vi "temporisador.vi"() -> ()   [LabVIEW 2020]
panel:
  in  "Auto Reset":bool=TRUE
  in  "Time Target (s)":dbl=1.0
  out "Numeric":i32
  in  "stop":bool
  in  "reset":bool
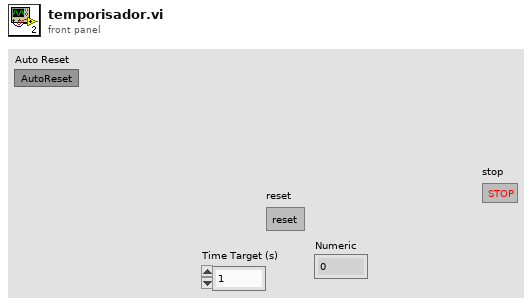
[diagram p1: front panel]
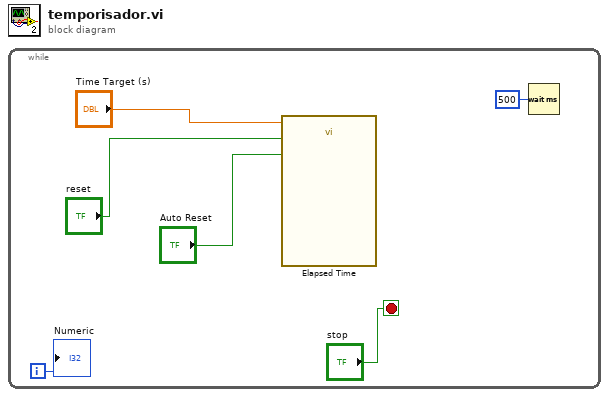
[diagram p0: block diagram]
diagram:
  n1 = while {
    i -> [w4]
    stop <- "stop" stop-if-true
    n2 = call "Elapsed Time"("Time Target (s)"="Time Target (s)", "Reset"="reset", "Auto Reset"="Auto Reset") -> ()  [unwired: 9 in, 8 out]
    n3 = Wait (ms)(milliseconds to wait=u32 500) -> ()  [unwired: 1 out]
    "Numeric" <- w4
  }
